vi "ConfigureTrig.vi"(8 "error in (no error)":errorcluster, 10 "TrigName":string, 11 "NiPxi6683H in":refnum<class "NiPxi6683H.lvclass">) -> (0 "error out":errorcluster, 3 "NiPxi6683H out":refnum<class "NiPxi6683H.lvclass">)   [LabVIEW 2014, in "SyncPlugins.lvlib" / "NiPxi6683H.lvclass"]
uses:
  NiPxi6683H.lvclass
  NiPxi6683H.lvclass/NiPxi6683H.ctl
  NiPxi6682/NiPxi6682.lvclass/NiPxi6682.ctl
  NiPxi6682/Accessors/Read NiSyncHandle.vi
  NiPxi6682/Accessors/Write NiSyncHandle.vi
  Accessors/Write Triggers.vi
  Accessors/Read Triggers.vi
  <vilib>/Utility/error.llb/Error Cluster From Error Code.vi
  <vilib>/ErrorRing/Error Ring.xnode
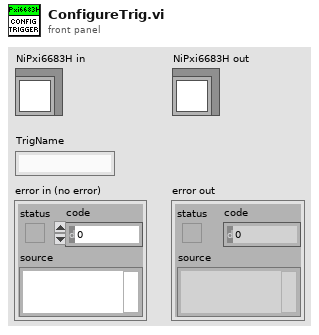
[diagram p1: front panel]
types:
  T1 = typedef "SyncPlugins.lvlib/PXI_MultiTrig.lvclass/clTrigger.ctl" = cluster{"Name":string, "DestTerm":string, "SrcTerm":string, "SyncClk":string, "Edge":i32, "Invert?":i32, "Initiated":bool, "Type":string, "TrigTime":bool}
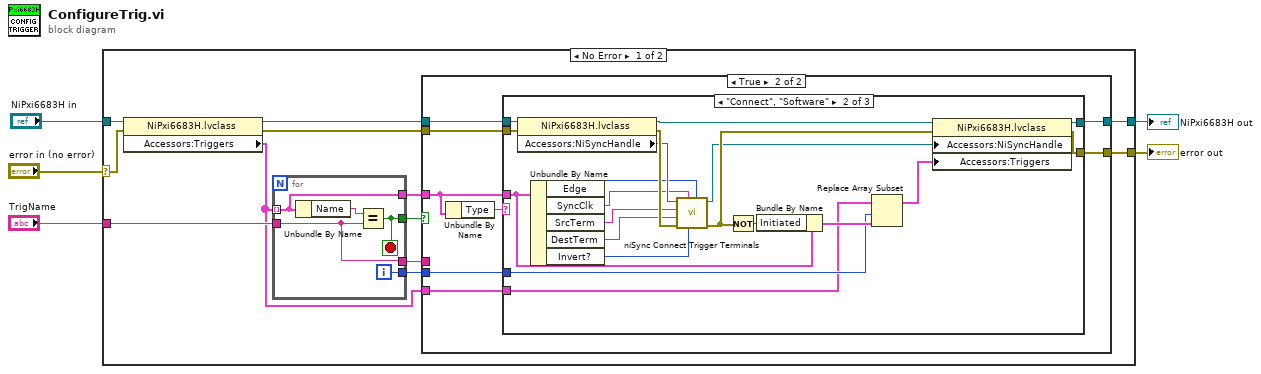
[diagram p0: block diagram]
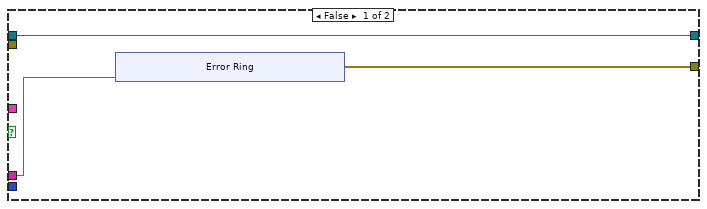
[diagram p2: hidden frame]
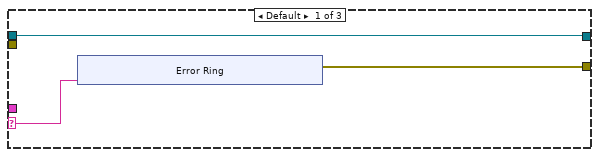
[diagram p3: hidden frame]
diagram:
  n1 = case shown="No Error" "error in (no error)" {
    selector: "error in (no error)" -> [w16 w73]
    tunnel: "NiPxi6683H in" -> [w17 w74]
    tunnel: "TrigName" -> [w15 _]
    tunnel: [w9 w73] -> w1
    tunnel: [w8 w74] -> w2
    frame No Error {
      n2 = property class="NiPxi6683H.lvclass"(reference=w17, error in=w16) -> (reference out=w11:refnum<class "NiPxi6683H.lvclass">, error out=w10:errorcluster, "Accessors:Triggers"=w7:T1[])
      n3 = for {
        tunnel: w7 -> [w72] mode=indexing
        tunnel: [w72] -> w12
        tunnel: w15 -> [w68]
        tunnel: [w70] -> w14
        tunnel: [w69] -> w13
        tunnel: [w68] -> w6
        i -> [w69]
        stop <- w70 stop-if-true
        n4 = Unbundle By Name(w72) -> ("Name"=w71:string)
        n5 = Equal?(x=w71, y=w68) -> (x = y?=w70:bool)
      }
      n6 = case shown="True" w14 {
        tunnel: w13 -> [_ w31]
        tunnel: w12 -> [_ w34]
        tunnel: w11 -> [w19 w32]
        tunnel: w10 -> [_ w33]
        tunnel: [w20 w30] -> w9
        tunnel: [w19 w28] -> w8
        tunnel: w7 -> [_ w29]
        tunnel: w6 -> [w18 _]
        frame False {
          n7 = xnode "Error Ring"("parameter 0"=w18) -> ("error out"=w20:errorcluster)
        }
        frame True {
          n8 = Unbundle By Name(w34) -> ("Type"=w35:string)
          n9 = case shown="\"Connect\", \"Software\"" w35 {
            selector: w35 -> [w38 _ _]
            tunnel: w34 -> [_ w60 _]
            tunnel: w33 -> [_ w65 w66]
            tunnel: w32 -> [w36 w64 w67]
            tunnel: w31 -> [_ w58 _]
            tunnel: [w37 w54 w66] -> w30
            tunnel: w29 -> [_ w57 _]
            tunnel: [w36 w55 w67] -> w28
            frame Default {
              n10 = xnode "Error Ring"("parameter 0"=w38) -> ("error out"=w37:errorcluster)
            }
            frame "Connect", "Software" {
              n11 = property class="NiPxi6683H.lvclass"(reference=w64, error in=w65) -> (reference out=w56:refnum<class "NiPxi6683H.lvclass">, error out=w63:errorcluster, "Accessors:NiSyncHandle"=w62:refnum<k15>)
              n12 = Unbundle By Name(w60) -> ("Edge"=w50:i32, "SyncClk"=w49:string, "SrcTerm"=w48:string, "DestTerm"=w47:string, "Invert?"=w46:i32)
              n13 = call <instrlib>:"niSync Connect Trigger Terminals.vi"("update edge (Rising Edge)"=w50, "invert (Don't Invert Signal)"=w46, "synchronization clock"=w49, "error in (no error)"=w63, "destination terminal"=w47, "source terminal"=w48, "instrument handle"=w62) -> ("error out"=w53:errorcluster, "instrument handle out"=w52:refnum<k15>)  [unwired: 3 in]
              n14 = Not(x=w53) -> (.not. x?=w61:bool)
              n15 = Bundle By Name(cluster=w60, "Initiated"=w61) -> (w59:T1)
              n16 = Replace Array Subset(array=w57, new element=w59, index=w58) -> (w51:T1[])
              n17 = property class="NiPxi6683H.lvclass"(reference=w56, error in=w53, "Accessors:NiSyncHandle"=w52, "Accessors:Triggers"=w51) -> (reference out=w55:refnum<class "NiPxi6683H.lvclass">, error out=w54:errorcluster)
            }
            frame "Timed" {
              # "Timed Triggers are configured by request.\nSee TimedTrigger.vi"
            }
          }
        }
      }
    }
    frame Error {
    }
  }
  "error out" <- w1
  "NiPxi6683H out" <- w2
